vi "P9374A NA set power.vi"(7 "Power dBm":dbl, 8 "error in (no error)":errorcluster {"code" format="%.0x"}, 11 "resource name":refnum<k15>="P9374A" caption="resource string") -> (0 "error out":errorcluster {"code" format="%.0x"}, 3 "instrument handle out":refnum<k15>)   [LabVIEW 2021]
uses:
  <instrlib>/Agilent NA/Agilent NA.lvlib
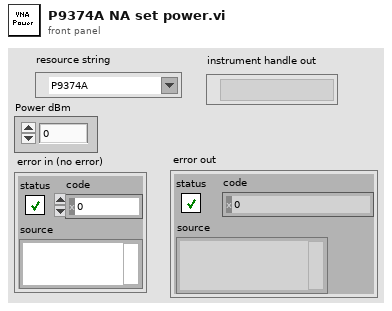
[diagram p1: front panel]
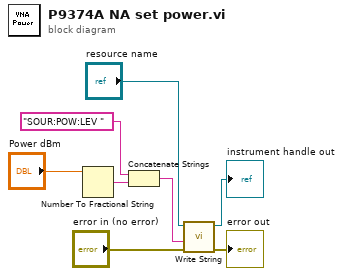
[diagram p0: block diagram]
diagram:
  n1 = Number To Fractional String(number="Power dBm") -> (F-format string=w5:string)  [unwired: 3 in]
  n2 = Concatenate Strings("SOUR:POW:LEV ", w5) -> (w4:string)
  n3 = call <instrlib>:"Write String.vi"("error in (no error)"="error in (no error)", "Command"=w4, "instrument handle"="resource name") -> ("error out"=→"error out":errorcluster, "instrument handle out"=→"instrument handle out":refnum<k15>)  [unwired: 7 in]
